vi "5802 Auto.vi"   [LabVIEW 2020]
uses:
  C:/Users/Nelson/Downloads/STEMateros/CompetionCode2022/Robot Global Data.vi
  <vilib>/Utility/file.llb/Read Delimited Spreadsheet (DBL).vi
  <vilib>/Rock Robotics/Network Tables/NT Read String.vi
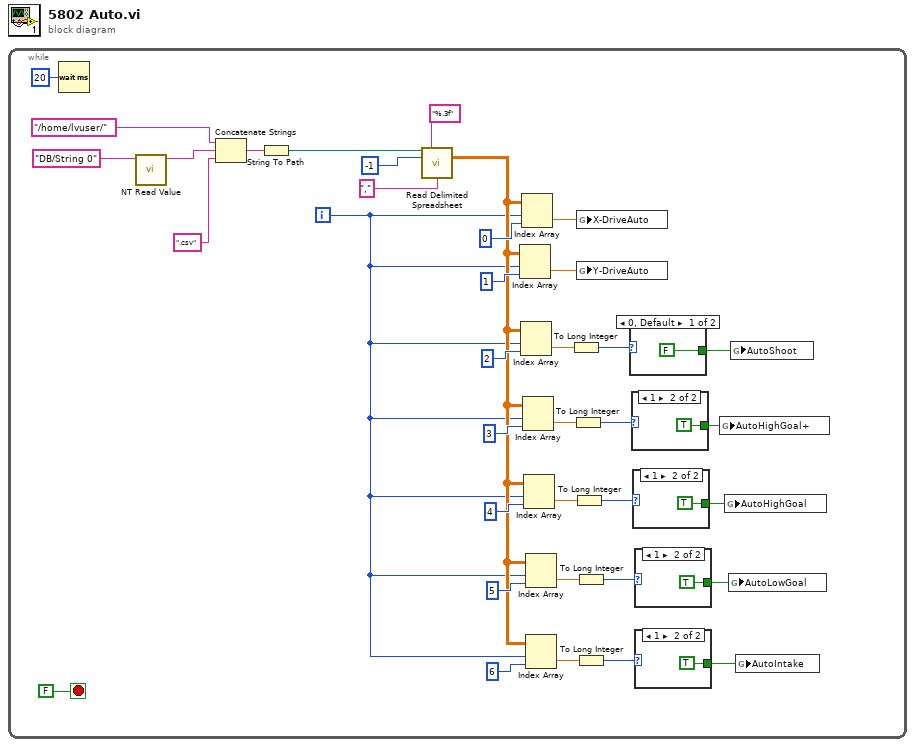
[diagram p0: block diagram]
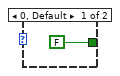
[diagram p2: hidden frame]
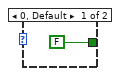
[diagram p3: hidden frame]
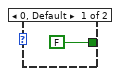
[diagram p4: hidden frame]
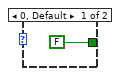
[diagram p5: hidden frame]
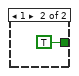
[diagram p6: hidden frame]
diagram:
  n1 = while {
    i -> [w7]
    stop <- FALSE stop-if-true
    n2 = Wait (ms)(milliseconds to wait=u32 20) -> ()  [unwired: 1 out]
    n3 = call-poly <vilib>:"NT Read Value.vi"("Name"="DB/String 0") -> ("String"=w4:string)  [unwired: 9 in, 1 out]
    n4 = Concatenate Strings("/home/lvuser/", w4, ".csv") -> (w2:string)
    n5 = String To Path(string=w2) -> (path=w1:path)
    n6 = call-poly <vilib>:"Read Delimited Spreadsheet.vi"("file path (dialog if empty)"=w1, "format (%.3f)"="%.3f", "number of rows (all:-1)"=-1, "delimiter (\\t)"="," ("delimiter (\\t)")) -> ("all rows"=w8:dbl[][])  [unwired: 6 in, 5 out]
    n7 = Index Array(array=w8, index (row)=w7, index (col)=1 ("disabled index (col)")) -> (element=w29:dbl)
    n8 = Index Array(array=w8, index (row)=w7, index (col)=2 ("disabled index (col)")) -> (element=w27:dbl)
    n9 = Index Array(array=w8, index (row)=w7, index (col)=0 ("disabled index (col)")) -> (element=w30:dbl)
    n10 = Index Array(array=w8, index (row)=w7, index (col)=3 ("disabled index (col)")) -> (element=w23:dbl)
    n11 = Index Array(array=w8, index (row)=w7, index (col)=4 ("disabled index (col)")) -> (element=w19:dbl)
    n12 = Index Array(array=w8, index (row)=w7, index (col)=5 ("disabled index (col)")) -> (element=w15:dbl)
    n13 = Index Array(array=w8, index (row)=w7, index (col)=6 ("disabled index (col)")) -> (element=w11:dbl)
    n14 = To Long Integer(number=w27) -> (32bit integer=w25:i32)
    n15 = To Long Integer(number=w23) -> (32bit integer=w21:i32)
    n16 = To Long Integer(number=w19) -> (32bit integer=w17:i32)
    n17 = To Long Integer(number=w15) -> (32bit integer=w13:i32)
    n18 = To Long Integer(number=w11) -> (32bit integer=w9:i32)
    n19 = global write "Robot Global Data.vi" "X-DriveAuto"(w30) -> ()
    n20 = global write "Robot Global Data.vi" "Y-DriveAuto"(w29) -> ()
    n21 = case shown="0, Default" w25 {
      tunnel: [FALSE TRUE] -> w26
      frame 0, Default {
      }
      frame 1 {
      }
    }
    n22 = case shown="1" w21 {
      tunnel: [FALSE TRUE] -> w22
      frame 0, Default {
      }
      frame 1 {
      }
    }
    n23 = case shown="1" w17 {
      tunnel: [FALSE TRUE] -> w18
      frame 0, Default {
      }
      frame 1 {
      }
    }
    n24 = case shown="1" w13 {
      tunnel: [FALSE TRUE] -> w14
      frame 0, Default {
      }
      frame 1 {
      }
    }
    n25 = case shown="1" w9 {
      tunnel: [FALSE TRUE] -> w10
      frame 0, Default {
      }
      frame 1 {
      }
    }
    n26 = global write "Robot Global Data.vi" "AutoHighGoal+"(w22) -> ()
    n27 = global write "Robot Global Data.vi" "AutoHighGoal"(w18) -> ()
    n28 = global write "Robot Global Data.vi" "AutoLowGoal"(w14) -> ()
    n29 = global write "Robot Global Data.vi" "AutoShoot"(w26) -> ()
    n30 = global write "Robot Global Data.vi" "AutoIntake"(w10) -> ()
  }
